vi "experiment-CoerseNumericType.vi"() -> ()   [LabVIEW 2019]
uses:
  <vilib>/Utility/Data Type/NI_Data Type.lvlib
panel:
  out "String":string
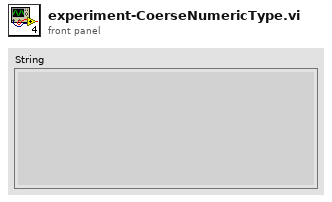
[diagram p1: front panel]
types:
  T1 = typedef "LVFixedPointRepBitsTypeDef.ctl" = cluster{"Signed":bool, "Word Length":u32, "Integer Word Length":i32}
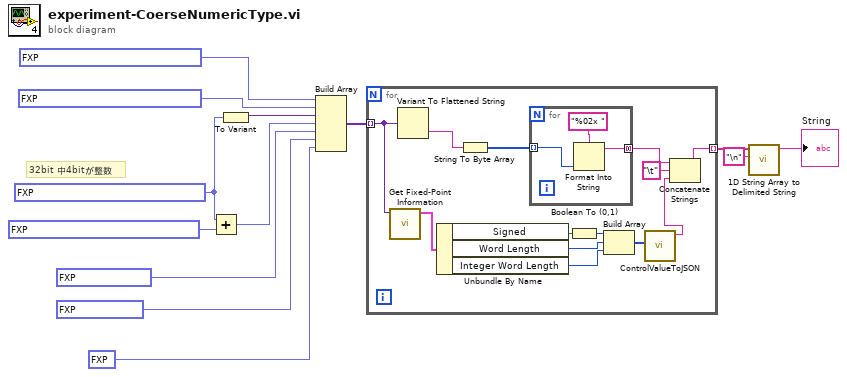
[diagram p0: block diagram]
diagram:
  w11 = fxp<+/-,32,4> data[16B] ("fixed-point type")
  # "32bit 中4bitが整数"
  n1 = Add(x=w11, y=fxp<+/-,32,4> data[16B]) -> (x+y=w9:fxp<+/-,32,4>)
  n2 = To Variant(anything=w11) -> (Variant=w10:variant)
  n3 = Build Array(fxp<+/-,32,4> -1.1000000014901161 ("fixed-point type"), fxp<+,32,4> 7.99999999627471 ("fixed-point type"), w10, w9, fxp<+/-,16,4> data[16B] ("y"), fxp<+/-,16,4> 7.999755859375 ("y"), fxp<+/-,4,2> 1.75 ("y")) -> (w8:variant[])
  n4 = for {
    tunnel: w8 -> [w24] mode=indexing
    tunnel: [w16] -> w13 mode=indexing
    n5 = call <vilib>:"Get Fixed-Point Information.vi"("variant"=w24) -> ("FXP representation"=w23:T1)  [unwired: 7 in, 3 out]
    n6 = Variant To Flattened String(Variant=w24) -> (data string=w26:string)  [unwired: 1 out]
    n7 = Unbundle By Name(w23) -> ("Signed"=w22:bool, "Word Length"=w20:u32, "Integer Word Length"=w19:i32)
    n8 = String To Byte Array(string=w26) -> (unsigned byte array=w25:u8[])
    n9 = for {
      tunnel: w25 -> [w29] mode=indexing
      tunnel: [w27] -> w17 mode=concatenating
      n10 = Format Into String(format string="%02x ", w29) -> (resulting string=w27:string)  [unwired: 2 in, 1 out]
    }
    n11 = Boolean To (0,1)(Boolean=w22) -> (0, 1=w21:i16)
    n12 = Build Array(w21, w20, w19) -> (w18:u32[])
    n13 = call "ControlValueToJSON.vi"("Value"=w18) -> ("String"=w14:string)  [unwired: 9 in, 1 out]
    n14 = Concatenate Strings(w17, "\t" ("string"), w14) -> (w16:string)
  }
  n15 = call <vilib>:"1D String Array to Delimited String.vi"("delimiter"="\n", "string array"=w13) -> ("delimited string"=→"String":string)  [unwired: 9 in]
